vi "create_full_token.vi"(8 "error in (no error)":errorcluster, 11 "llm_openai_chatmodels in":refnum<class "llm_openai_chatmodels.lvclass">) -> (0 "error out":errorcluster, 1 "token":string, 2 "header":string(combo)="Authorization", 3 "llm_openai_chatmodels out":refnum<class "llm_openai_chatmodels.lvclass">)   [LabVIEW 2020, in "llm_openai_chatmodels.lvclass"]
uses:
  llm_openai_chatmodels.lvclass
  llm_openai_chatmodels.lvclass/llm_openai_chatmodels.ctl
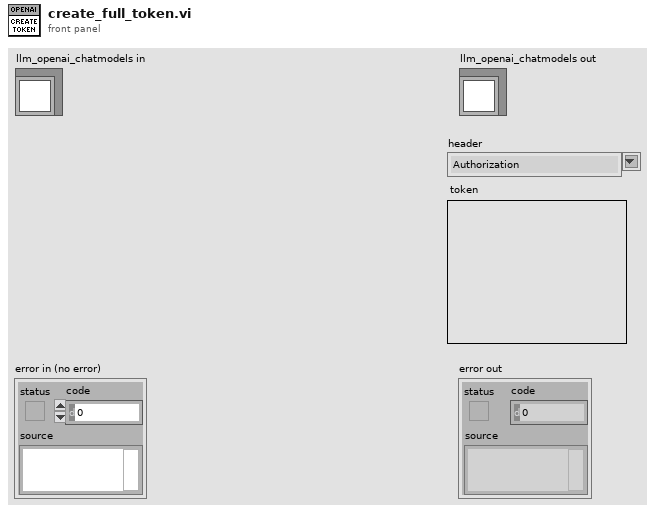
[diagram p1: front panel]
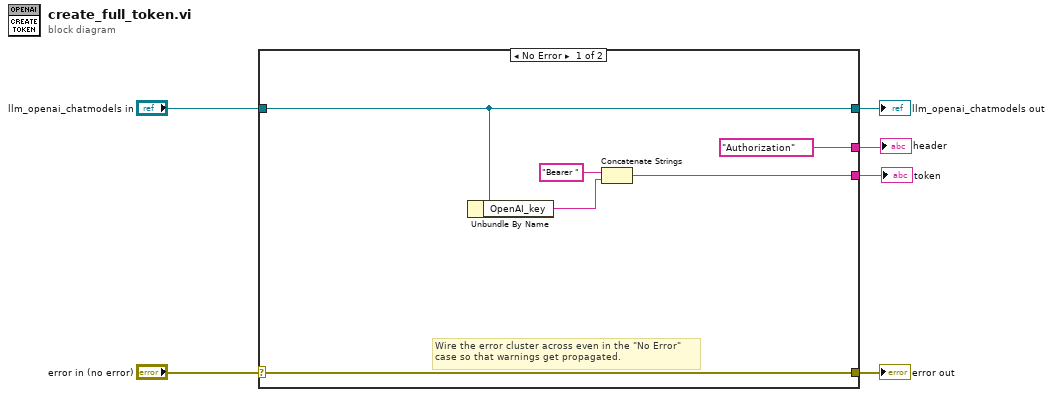
[diagram p0: block diagram]
diagram:
  n1 = case shown="No Error" "error in (no error)" {
    selector: "error in (no error)" -> [w12 w14]
    tunnel: [w12 w14] -> w5
    tunnel: [w11 w13] -> w3
    tunnel: "llm_openai_chatmodels in" -> [w11 w13]
    tunnel: [w8 _] -> w2
    tunnel: ["Authorization" ("header") _] -> w1
    frame No Error {
      # "Wire the error cluster across even in the \"No Error\"\ncase so that warnings get propagated."
      n2 = Unbundle By Name(w11) -> ("OpenAI_key"=w9:string)
      n3 = Concatenate Strings("Bearer " ("value"), w9) -> (w8:string)
    }
    frame Error {
    }
  }
  "error out" <- w5
  "llm_openai_chatmodels out" <- w3
  "token" <- w2
  "header" <- w1
